vi "Username&Password.vi"() -> ()   [LabVIEW 2012]
uses:
  <vilib>/addons/database/NI_Database_API.lvlib
  <vilib>/addons/database/Connection.llb/DB Tools Open Connec (Path).vi
  <vilib>/addons/database/Connection.llb/Conn Execute.vi
  <vilib>/addons/database/Recordset.llb/Rec Destroy - Connection.vi
panel:
  in  "Password":string
  in  "Username":string
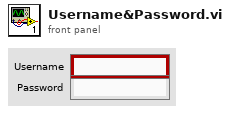
[diagram p1: front panel]
types:
  T1 = typedef "NI_Database_API.lvlib/Conn ObjectReference.ctl" = refnum<k1>
  T2 = typedef "NI_Database_API.lvlib/Rec ObjectReference.ctl" = refnum<k1>
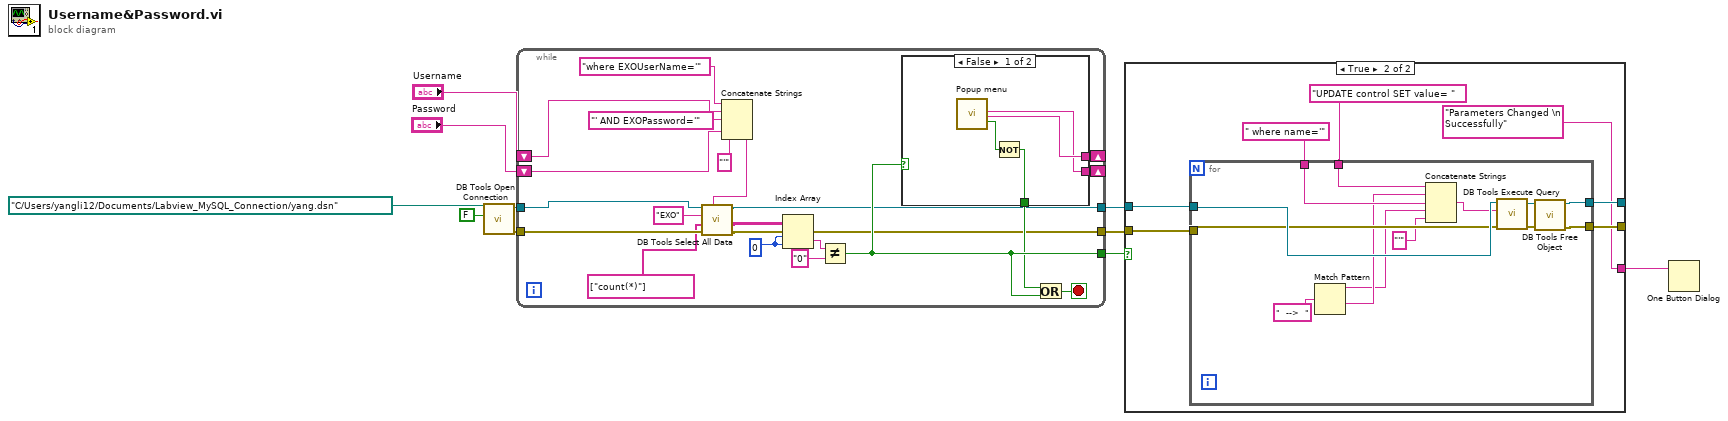
[diagram p0: block diagram]
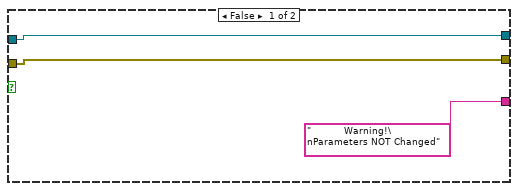
[diagram p2: hidden frame]
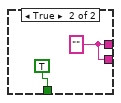
[diagram p3: hidden frame]
diagram:
  n1 = call-poly <vilib>:"DB Tools Open Connection.vi"("prompt? (F)"=FALSE, "connection information"=path "C:/Users/yangli12/Documents/Labview_MySQL_Connection/yang.dsn") -> ("error out"=w10:errorcluster, "connection reference"=w9:T1)  [unwired: 6 in]
  n2 = while {
    tunnel: w10 -> [w15]
    tunnel: w9 -> [w17]
    tunnel: [w12] -> w4
    tunnel: [w14] -> w3
    tunnel: [w24] -> w2
    shift-right: [w22] -> _
    shift-left: "Username" -> [w20]
    shift-right: [w21] -> _
    shift-left: "Password" -> [w19]
    stop <- w25 stop-if-true
    w27 = 0 ("disabled index (col)")
    n3 = Concatenate Strings("where EXOUserName='" ("string"), w20, "' AND EXOPassword='" ("string"), w19, "'" ("string")) -> (w18:string)
    n4 = call <vilib>:"DB Tools Select All Data.vi"("optional clause"=w18, "error in (no error)"=w15, "columns"=string[] ["count(*)"], "table"="EXO", "connection reference"=w17) -> ("error out"=w14:errorcluster, "data"=w13:string[][], "connection reference out"=w12:T1)  [unwired: 1 in]
    n5 = Index Array(array=w13, index (row)=w27, index (col)=w27) -> (element=w28:string)
    n6 = Not Equal?(x=w28, y="0") -> (x != y?=w24:bool)
    n7 = case shown="False" w24 {
      tunnel: [w32 TRUE ("T button?")] -> w23
      tunnel: [w35 w36] -> w22
      tunnel: [w34 w36] -> w21
      frame False {
        n8 = call "Popup menu.vi"() -> ("Password"=w34:string, "Username"=w35:string, "Retry"=w33:bool)  [unwired: 16 in, 1 out]
        n9 = Not(x=w33) -> (.not. x?=w32:bool)
      }
      frame True {
        w36 = "" ("Username")
      }
    }
    n10 = Or(x=w23, y=w24) -> (x .or. y?=w25:bool)
  }
  n11 = case shown="True" w2 {
    tunnel: [w40 w45] -> _
    tunnel: [w39 w44] -> _
    tunnel: w4 -> [w40 w43]
    tunnel: w3 -> [w39 w42]
    tunnel: ["           Warning!\nParameters NOT Changed" "Parameters Changed \n        Successfully"] -> w1
    frame False {
    }
    frame True {
      n12 = for {
        tunnel: w43 -> [w59]
        tunnel: w42 -> [w58]
        tunnel: "UPDATE control SET value= " -> [w60]
        tunnel: [w57] -> w45
        tunnel: [w56] -> w44
        tunnel: " where name='" ("string") -> [w55]
        n13 = Match Pattern(regular expression="  -->  ") -> (before substring=w48:string, after substring=w50:string)  [unwired: 2 in, 2 out]
        n14 = Concatenate Strings(w60, w50, w55, w48, "'" ("string")) -> (w54:string)
        n15 = call-poly <vilib>:"DB Tools Execute Query.vi"("error in (no error)"=w58, "SQL query"=w54, "connection reference"=w59) -> ("error out"=w52:errorcluster, "recordset reference"=w53:T2)  [unwired: 5 in]
        n16 = call-poly <vilib>:"DB Tools Free Object.vi"("error in (no error)"=w52, "recordset reference"=w53) -> ("error out"=w56:errorcluster, "connection reference"=w57:T1)  [unwired: 8 in]
      }
    }
  }
  n17 = One Button Dialog(message=w1) -> ()  [unwired: 1 in, 1 out]
